vi "Read Programmer Details.vi"(8 "error in":errorcluster, 11 "MPLab in":refnum<class "MPLab.lvclass">) -> (0 "error out":errorcluster, 3 "MPLab out":refnum<class "MPLab.lvclass">)   [LabVIEW 2018, in "MPLab.lvlib" / "MPLab.lvclass"]
uses:
  MPLab.lvclass
  MPLab.lvclass/MPLab.ctl
  builds/Flash Utility.lvlibp/Flash Utility.lvclass
  builds/Configuration.lvlibp/Configuration.lvclass
  C:/Users/Ron.Dexter.LUMINARTECH/Desktop/builds/Flash Utility.lvlibp/Flash Utility.lvclass
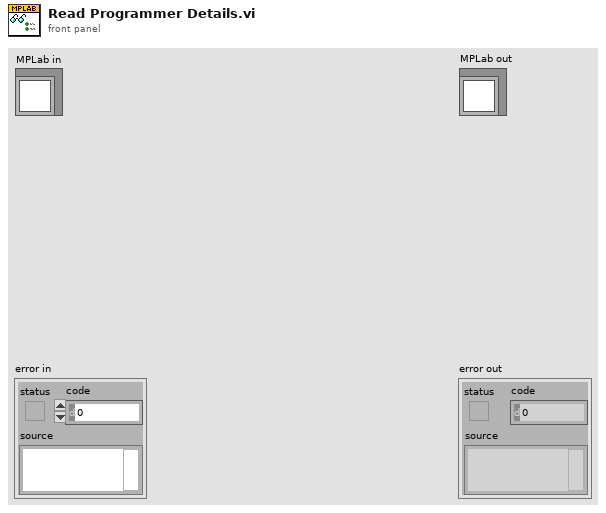
[diagram p1: front panel]
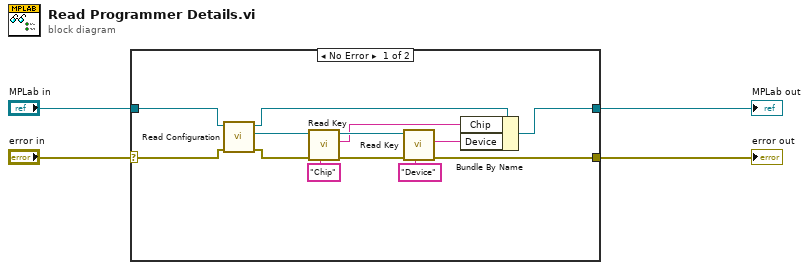
[diagram p0: block diagram]
diagram:
  n1 = case shown="No Error" "error in" {
    selector: "error in" -> [w6 w19]
    tunnel: [w5 w19] -> w3
    tunnel: [w13 w18] -> w1
    tunnel: "MPLab in" -> [w10 w18]
    frame No Error {
      n2 = call "Read Configuration.vi"("error in (no error)"=w6, "Flash Utility in"=w10) -> ("error out"=w8:errorcluster, "Configuration"=w16:refnum<class "Configuration.lvclass">, "Flash Utility out"=w9:refnum<class "MPLab.lvclass">)  [unwired: 7 in]
      n3 = call "Read Key.vi"("Key:"="Chip", "error in"=w8, "Configuration in"=w16) -> ("error out"=w7:errorcluster, "Value"=w11:string, "Configuration out"=w17:refnum<class "Configuration.lvclass">)  [unwired: 6 in]
      n4 = call "Read Key.vi"("Key:"="Device", "error in"=w7, "Configuration in"=w17) -> ("error out"=w5:errorcluster, "Value"=w12:string)  [unwired: 6 in, 1 out]
      n5 = Bundle By Name(cluster=w9, "Chip"=w11, "Device"=w12) -> (w13:refnum<class "MPLab.lvclass">)
    }
    frame Error {
    }
  }
  "error out" <- w3
  "MPLab out" <- w1
